vi "Stage_FGV.vi"(6 "Operation(Read)":enum16{"Write", "Read"}(ring)=enum."Read", 8 "error in (no error)":errorcluster, 11 "reference in":refnum<k24>) -> (0 "error out":errorcluster, 3 "reference out":refnum<k24>)   [LabVIEW 2020]
uses:
  C:/Users/MarcuLab/Desktop/V6 APD LV/V6 APD LV/Kinesis/ThorLabs.MotionControl.KCube.DCServoCLI.dll
  Kinesis/ThorLabs.MotionControl.KCube.DCServoCLI.dll
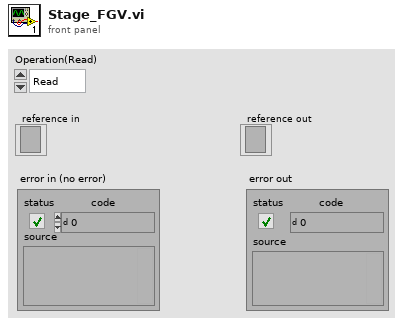
[diagram p1: front panel]
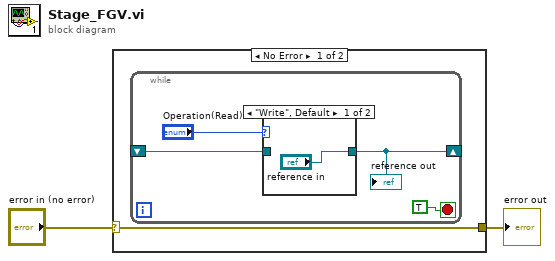
[diagram p0: block diagram]
diagram:
  n1 = case shown="No Error" "error in (no error)" {
    selector: "error in (no error)" -> [w3 w10]
    tunnel: [w3 w10] -> w1
    frame No Error {
      n2 = while {
        shift-right: [w5] -> _
        shift-left: _ -> [w4]
        stop <- TRUE stop-if-true
        n3 = case shown="\"Write\", Default" "Operation(Read)" {
          tunnel: ["reference in" w9] -> w5
          tunnel: w4 -> [_ w9]
          frame "Write", Default {
          }
          frame "Read" {
          }
        }
        "reference out" <- w5
      }
    }
    frame Error {
    }
  }
  "error out" <- w1
